vi "FunctAcq_Generate single POI timestamps.vi"(6 "ROI number":i32, 7 "Number of data points in single POI (all trials)":i32, 9 "Funct Acq cycle length (us)":dbl, 10 "Single funct.acq cycle time-stamps (us)":dbl[](array[numeric])) -> (3 "Full timestamps array for single POI (sec)":sgl[](array[numeric]))   [LabVIEW 2020]
panel:
  out "Output points":i32
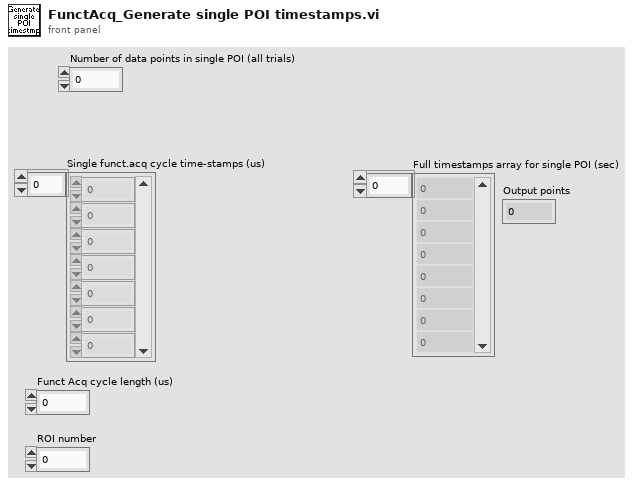
[diagram p1: front panel]
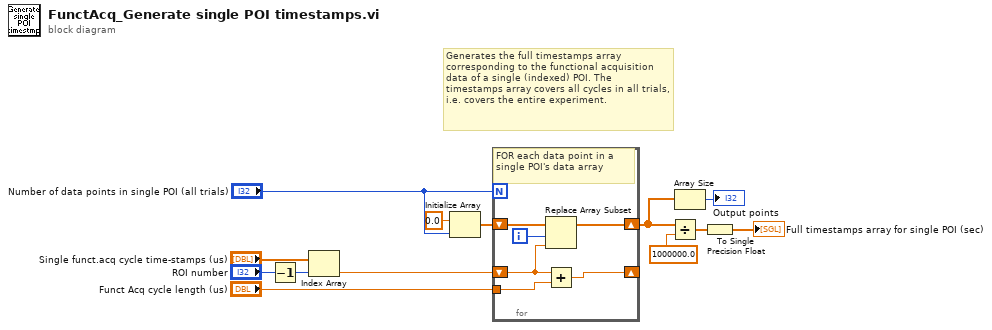
[diagram p0: block diagram]
diagram:
  # "Generates the full timestamps array corresponding to the functional acquisition data of a single (indexed) POI. The timestamps array covers all cycles in all trials, i.e. covers the entire experiment."
  n1 = Decrement(x="ROI number") -> (x-1=w5:i32)
  n2 = Index Array(array="Single funct.acq cycle time-stamps (us)", index=w5) -> (element=w9:dbl)
  n3 = Initialize Array(0.0 ("element"), "Number of data points in single POI (all trials)") -> (w12:dbl[])
  n4 = for {
    N: "Number of data points in single POI (all trials)" -> [_]
    shift-right: [w17] -> w4
    shift-left: w12 -> [w19]
    shift-right: [w15] -> _
    shift-left: w9 -> [w16]
    tunnel: "Funct Acq cycle length (us)" -> [w14]
    i -> [w18]
    # "FOR each data point in a single POI's data array"
    n5 = Replace Array Subset(array=w19, new element=w16, index=w18) -> (w17:dbl[])
    n6 = Add(x=w16, y=w14) -> (x+y=w15:dbl)
  }
  n7 = Divide(x=w4, y=1000000.0) -> (x/y=w3:dbl[])
  n8 = Array Size(array=w4) -> (size(s)=→"Output points":i32)
  n9 = To Single Precision Float(number=w3) -> (single precision float=→"Full timestamps array for single POI (sec)":sgl[])
